vi "Initialize.vi"(0 "instruction target":refnum<class "niInstr FIFO Register Bus v1 Host.lvclass">, 1 "Sampling Info":T2={"Number of Channels"=4, "Actual Samp Rate"=4.0, "Chan Name Array"=[], "EU Chan Array"=[], "dB Ref Chan Array"=[]}, 5 "context":refnum<class "niInstr Instruction Framework Context v1 Host.lvclass">, 7 "FIFOs":T1, 11 "error in (no error)":errorcluster, 12 "instance":u8) -> (4 "task":refnum<class "WaveformTask.lvclass">, 15 "error out":errorcluster)   [LabVIEW 2015]
uses:
  WaveformTask.lvclass
  <instrlib>/_niInstr/FIFO Register Bus/v1/Host/niInstr FIFO Register Bus v1 Host.lvclass
  <instrlib>/_niInstr/Instruction Framework/v1/Host/Instruction Framework Context/niInstr Instruction Framework Context v1 Host.lvclass
  <vilib>/NI/cRIO Wfm/SamplingInfo.ctl
  <vilib>/NI/cRIO Wfm/cRIO Wfm.lvlib
  DataFIFOs.ctl
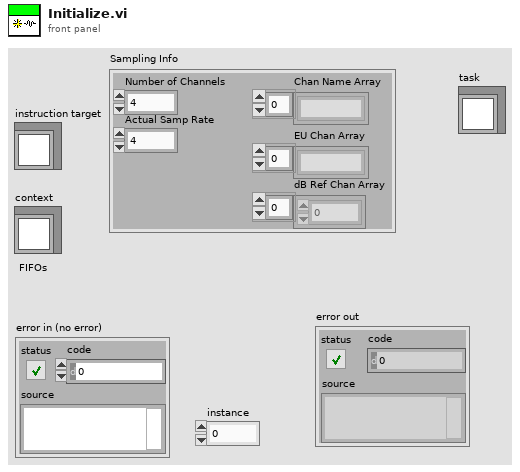
[diagram p1: front panel]
types:
  T1 = typedef "WaveformTask.lvclass/DataFIFOs.ctl" = refnum<k20>
  T2 = typedef "cRIO Wfm.lvlib/SamplingInfo.ctl" = cluster{"Number of Channels":i32, "Actual Samp Rate":dbl, "Chan Name Array":string[], "EU Chan Array":string[], "dB Ref Chan Array":dbl[]}
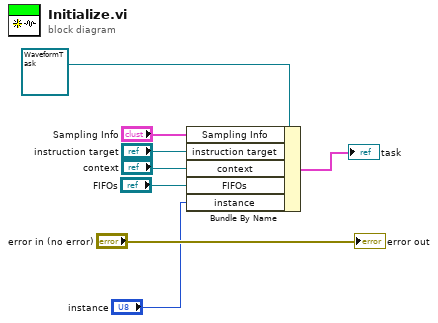
[diagram p0: block diagram]
diagram:
  n1 = Bundle By Name(cluster=refnum<class "WaveformTask.lvclass"> refnum ("WaveformAPI.lvlib:Task.lvclass"), "Sampling Info"="Sampling Info", "instruction target"="instruction target", "context"="context", "FIFOs"="FIFOs", "instance"="instance") -> (→"task":cluster{})
  "error out" <- "error in (no error)"
